vi "Determine Camera Type.vi"(9 "Camera Name":string, 11 "Robot IP":string) -> (0 "Camera Name":string, 1 "Camera Type":enum16{"None", "USB", "IP"}(ring), 2 "port":i32, 3 "address":string, 4 "cgi string":string)   [LabVIEW 2020]
uses:
  <vilib>/Rock Robotics/Network Tables/NT Read String Array.vi
  <vilib>/Rock Robotics/Network Tables/NT Read String.vi
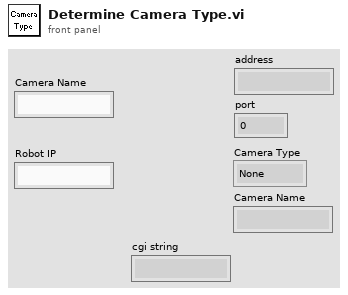
[diagram p1: front panel]
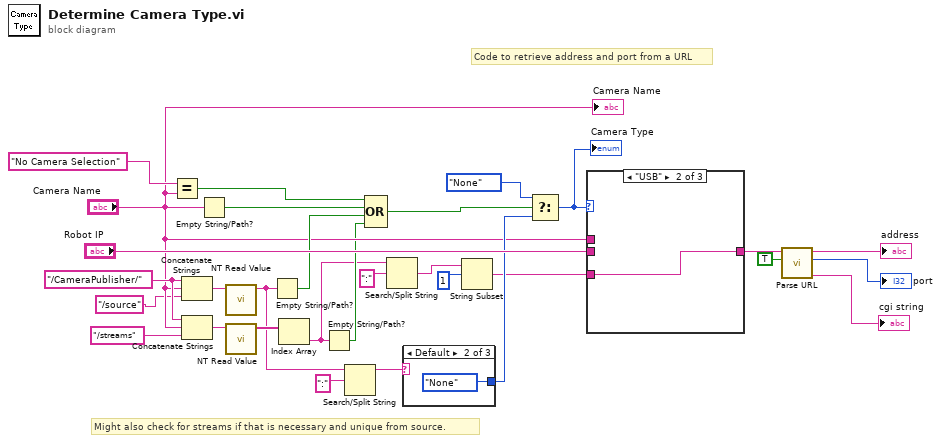
[diagram p0: block diagram]
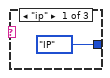
[diagram p2: hidden frame]
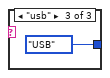
[diagram p3: hidden frame]
diagram:
  w20 = "/CameraPublisher/"
  # "Code to retrieve address and port from a URL"
  # "Might also check for streams if that is necessary and unique from source."
  n1 = Equal?(x="No Camera Selection", y="Camera Name") -> (x = y?=w26:bool)
  n2 = Concatenate Strings(w20, "Camera Name", "/source") -> (w23:string)
  n3 = Concatenate Strings(w20, "Camera Name", "/streams") -> (w18:string)
  n4 = Empty String/Path?(string/path="Camera Name") -> (empty?=w25:bool)
  n5 = call-poly <vilib>:"NT Read Value.vi"("Name"=w23) -> ("String"=w2:string)  [unwired: 9 in, 1 out]
  n6 = call-poly <vilib>:"NT Read Value.vi"("Name"=w18) -> ("String Array"=w14:string[])  [unwired: 9 in, 1 out]
  n7 = Empty String/Path?(string/path=w2) -> (empty?=w22:bool)
  n8 = Index Array(array=w14) -> (element=w8:string)  [unwired: 1 in]
  n9 = Empty String/Path?(string/path=w8) -> (empty?=w17:bool)
  n10 = Search/Split String(string=w2, search string/char (-)=":" ("format string")) -> (substring before match=w1:string)  [unwired: 1 in, 2 out]
  n11 = Compound Arithmetic op=OR(w26, w25, w22, w17) -> (w24:bool)
  n12 = Search/Split String(string=w8, search string/char (-)=":" ("format string")) -> (match + rest of string=w6:string)  [unwired: 1 in, 2 out]
  n13 = case shown="Default" w1 {
    tunnel: [enum16{"None", "USB", "IP"}."IP" ("Enum") enum16{"None", "USB", "IP"}."None" ("Enum") enum16{"None", "USB", "IP"}."USB" ("Enum")] -> w21
    frame "ip" {
    }
    frame Default {
    }
    frame "usb" {
    }
  }
  n14 = String Subset(string=w6, offset (0)=1) -> (substring=w4:string)  [unwired: 1 in]
  n15 = Select(t=enum16{"None", "USB", "IP"}."None" ("Enum"), s=w24, f=w21) -> (s? t:f=w29:enum16{"None", "USB", "IP"})
  "Camera Type" <- w29
  n16 = case shown="\"USB\"" w29 {
    tunnel: [w34 w35 w36] -> w12
    tunnel: "Robot IP" -> [_ _ _]
    tunnel: "Camera Name" -> [w34 _ _]
    tunnel: w4 -> [_ w35 w36]
    frame "None", Default {
    }
    frame "USB" {
    }
    frame "IP" {
    }
  }
  n17 = call "Parse URL.vi"("Full"=TRUE, "URL"=w12) -> ("cgi string"=→"cgi string":string, "port"=→"port":i32, "address"=→"address":string)  [unwired: 6 in, 1 out]
  "Camera Name" <- "Camera Name"
